vi "Set Tree Symbols.vi"(8 "error in (no error)":errorcluster, 11 "Test Executive View in":refnum<class "Test Executive View.lvclass">) -> (0 "error out":errorcluster, 3 "Test Executive View out":refnum<class "Test Executive View.lvclass">)   [LabVIEW 2019, in "Test Executive View.lvclass"]
uses:
  <vilib>/gpm_packages/@cs/Test-executive-builder/Example/Application/Test Executive View/Test Executive View/Test Executive View.lvclass
  C:/Program Files/National Instruments/LabVIEW 2019/vi.lib/gpm_packages/@cs/Test-executive-builder/Source/Test Executive Builder View/Test Executive Builder View/Test Executive Builder View.lvclass
  <vilib>/gpm_packages/@cs/Test-executive-builder/Source/Test Executive Builder View/Test Executive Builder View/Test Executive Builder View.lvclass/Test Executive Builder View.ctl
  <vilib>/gpm_packages/@cs/Test-executive-builder/Source/Test Executive Builder View/Test Executive Builder View/Test Executive Builder View.lvclass
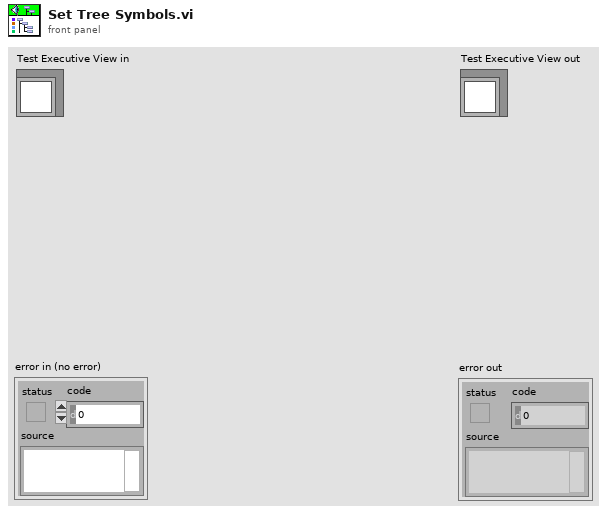
[diagram p1: front panel]
types:
  T1 = typedef "Tree Symbol.ctl" = cluster{"Index":i32, "Image":T2}
  T2 = typedef "imagedata.ctl" = cluster{"image type":i32, "image depth":i32, "image":u8[], "mask":u8[], "colors":u32[], "Rectangle":cluster{"left":i16, "top":i16, "right":i16, "bottom":i16}}
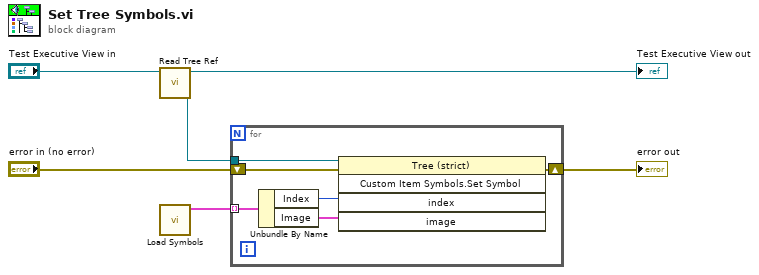
[diagram p0: block diagram]
diagram:
  n1 = call <vilib>:"Read Tree Ref.vi"("Test Executive Builder View in"="Test Executive View in") -> ("Tree Ref"=w6:refnum<vi>, "Test Executive Builder View out"=→"Test Executive View out":refnum<class "Test Executive View.lvclass">)  [unwired: 9 in]
  n2 = call <vilib>:"Load Symbols.vi"() -> ("Symbols"=w1:T1[])  [unwired: 11 in]
  n3 = for {
    tunnel: w6 -> [w12]
    tunnel: w1 -> [w11] mode=indexing
    shift-right: [w7] -> w2
    shift-left: "error in (no error)" -> [w8]
    n4 = Unbundle By Name(w11) -> ("Index"=w10:i32, "Image"=w9:T2)
    n5 = invoke class="Tree (strict)" method="Custom Item Symbols.Set Symbol"(reference=w12, error in=w8, "index"=w10, "image"=w9) -> (error out=w7:errorcluster)  [unwired: 1 in, 4 out]
  }
  "error out" <- w2
